vi "GetText.vi"(8 "error in":errorcluster, 11 "ScaleAndLimitModule editor node in":refnum<class "ScaleAndLimitModule editor node.lvclass">) -> (0 "error out":errorcluster, 1 "additional text":string, 2 "text":string, 3 "ScaleAndLimitModule editor node out":refnum<class "ScaleAndLimitModule editor node.lvclass">, 4 "glyph":string)   [LabVIEW 2017, in "ScaleAndLimitModule editor node.lvclass"]
uses:
  ScaleAndLimitModule editor node.lvclass
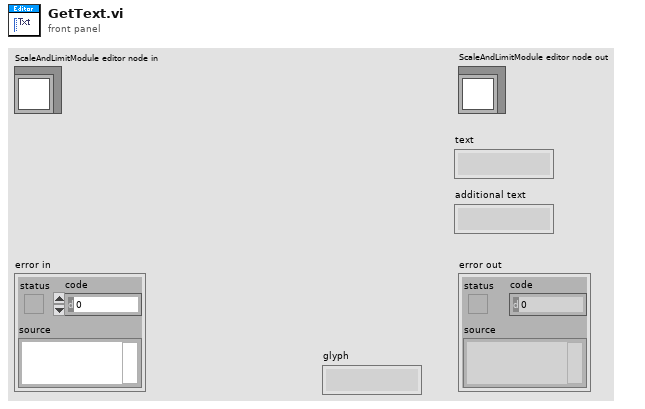
[diagram p1: front panel]
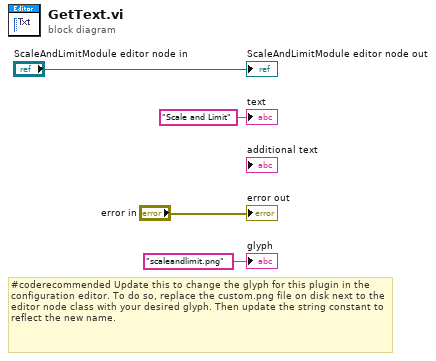
[diagram p0: block diagram]
diagram:
  # "#coderecommended Update this to change the glyph for this plugin in the configuration editor. To do so, replace the custom.png file on disk next to the editor node class with your desired glyph. Then update the string constant to reflect the new name."
  "error out" <- "error in"
  "ScaleAndLimitModule editor node out" <- "ScaleAndLimitModule editor node in"
  "text" <- "Scale and Limit" ("text")
  "glyph" <- "scaleandlimit.png" ("glyph")
